vi "Create.vi"(8 "error in (no error)":errorcluster) -> (0 "error out":errorcluster, 3 "CodeCoverage out":refnum<class "CodeCoverage.lvclass">)   [LabVIEW 2019, in "CodeCoverage.lvclass"]
doc: "Creates a new application instance for code coverage analysis."
uses:
  CodeCoverage.lvclass
  CodeCoverage.lvclass/CodeCoverage.ctl
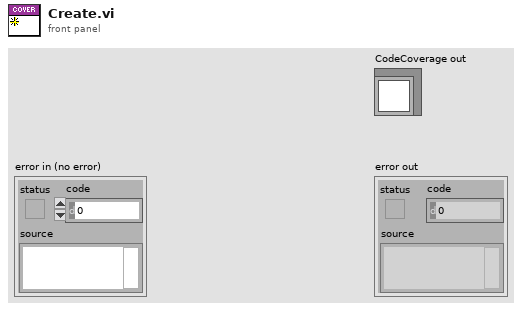
[diagram p1: front panel]
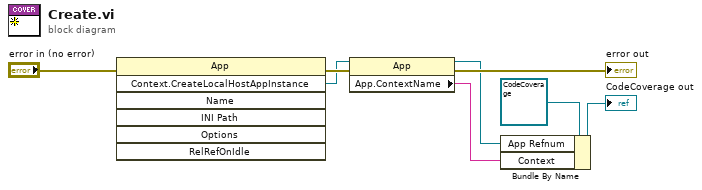
[diagram p0: block diagram]
diagram:
  n1 = invoke class="App" method="Context.CreateLocalHostAppInstance"(error in="error in (no error)") -> (error out=w6:errorcluster, "Create Context"=w5:refnum<vi>)  [unwired: 6 in, 5 out]
  n2 = property class="App"(reference=w5, error in=w6) -> (reference out=w1:refnum<vi>, error out=→"error out":errorcluster, "App.ContextName"=w4:string)
  n3 = Bundle By Name(cluster=refnum<class "CodeCoverage.lvclass"> refnum ("CodeCoverage in"), "App Refnum"=w1, "Context"=w4) -> (→"CodeCoverage out":refnum<class "CodeCoverage.lvclass">)
